vi "Query Counter presets.vi"(8 "error in (no error)":errorcluster, 10 "Counter (Def: T)":T1=enum."Counter T", 11 "VISA resource name":refnum<visa-resource-name>) -> (0 "error out":errorcluster, 2 "Number of triggers":dbl, 3 "VISA resource name out":refnum<visa-resource-name>)   [LabVIEW 2011, in "SR400.lvlib"]
doc: "CP i { ,n }\nThe CP command sets and reads the counter\npresets. If i = 1 then counter B is selected, if i = 2\ncounter T is selected. The parameter i is required.\nIf n is included, then counter i is preset to n where\nn is a value from 1 to 9E11. n may be expressed in\nany format but must be greater than or equal to 1\nand only the most significant digit is used. For\nexample, \"CP2,10\" , \"CP2,1E1\" , \"CP2,0.1E2\" ,\n\"CP2,12\" all set T SET to 1E1. Changing a\ncounter preset while counting causes the counters\nto pause. A counter start command or keypress\nresumes counting. If n is absent, then the preset\nvalue of counter i is returned. In the above\nexample, the string \"1E1\" is returned. Note that n\nis the number of cycles of the 10 MHz clock, not\nseconds."
uses:
  SR400.lvlib
  Typedefs/Counter Preset.ctl
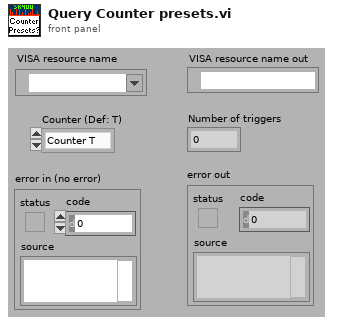
[diagram p1: front panel]
types:
  T1 = typedef "SR400.lvlib/Counter Preset.ctl" = enum16{"Invalid", "Counter B", "Counter T"}
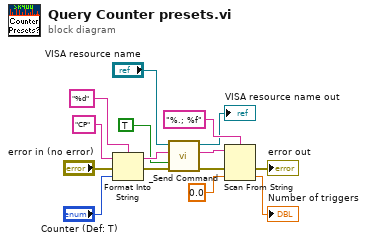
[diagram p0: block diagram]
diagram:
  n1 = Format Into String(format string="%d", initial string="CP" ("command"), error in="error in (no error)", "Counter (Def: T)") -> (resulting string=w6:string, error out=w5:errorcluster)
  n2 = call "_Send Command.vi"("error in (no error)"=w5, "Query? (F)"=TRUE, "Command"=w6, "VISA resource name"="VISA resource name") -> ("error out"=w2:errorcluster, "Response"=w3:string, "VISA resource name out"=→"VISA resource name out":refnum<visa-resource-name>)  [unwired: 5 out]
  n3 = Scan From String(format string="%.; %f", input string=w3, error in=w2, default 1=0.0 ("default value 1")) -> (error out=→"error out":errorcluster, output 1=→"Number of triggers":dbl)  [unwired: 1 in, 2 out]
